vi "Write VI path.vi"(8 "error in":errorcluster, 10 "VI path":path, 11 "UI Reference configuration in":refnum<class "io configuration.lvclass">) -> (0 "error out":errorcluster, 3 "UI Reference configuration out":refnum<class "io configuration.lvclass">)   [LabVIEW 2014, in "io configuration.lvclass"]
uses:
  io configuration.lvclass
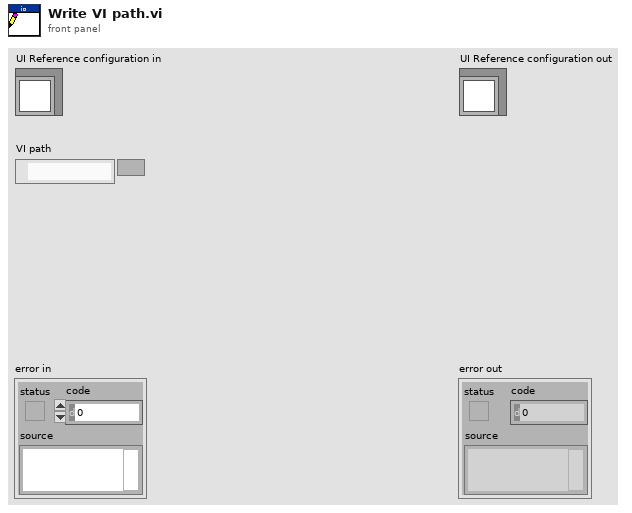
[diagram p1: front panel]
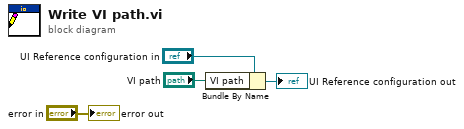
[diagram p0: block diagram]
diagram:
  n1 = Bundle By Name(cluster="UI Reference configuration in", "VI path"="VI path") -> (→"UI Reference configuration out":refnum<class "io configuration.lvclass">)
  "error out" <- "error in"
